vi "Set_valves.vi"() -> ()   [LabVIEW 2016]
panel:
  in  "Clean Cycle Wait Time (s)":u32=8
  in  "Clean Cycle":bool
  in  "Close all Valves":bool
  in  "Set new Values":bool
  in  "stop":bool
  in  "Update Immediately":bool=TRUE
  in  "Which box":string[](array[string])=["A", "B", "C"]
  in  "Channel Nums":string[](array[string])=["1", "2", "3", "4", "5", "6", "7", "8"]
  in  "Channels":bool[][](array[boolean])=[[FALSE, FALSE, FALSE], [FALSE, FALSE, FALSE], [FALSE, FALSE, FALSE], [FALSE, FALSE, FALSE], [FALSE, FALSE, FALSE], [FALSE, FALSE, FALSE], [FALSE, FALSE, FALSE], [FALSE, FALSE, FALSE]]
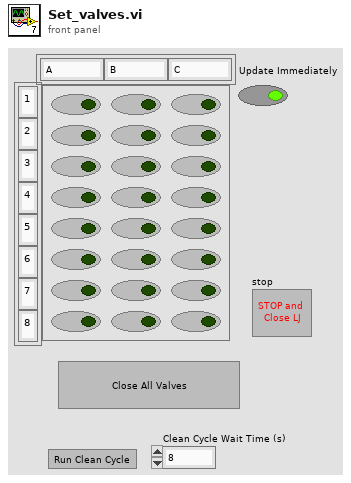
[diagram p1: front panel]
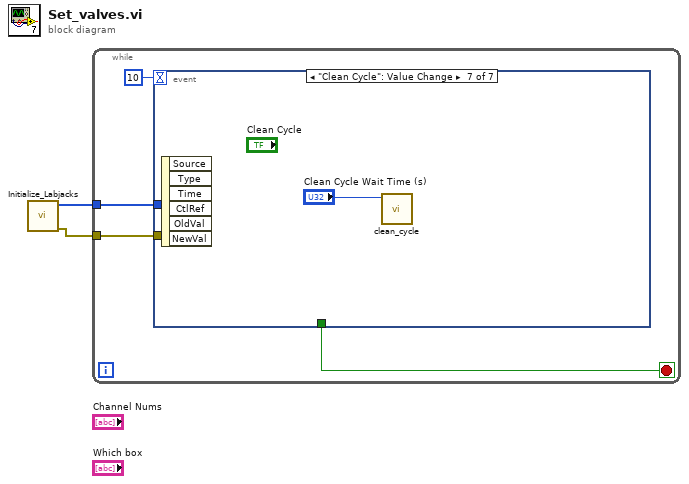
[diagram p0: block diagram]
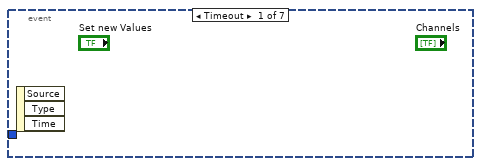
[diagram p2: hidden frame]
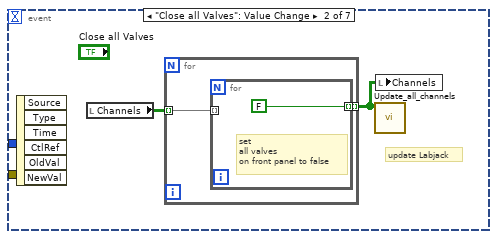
[diagram p3: hidden frame]
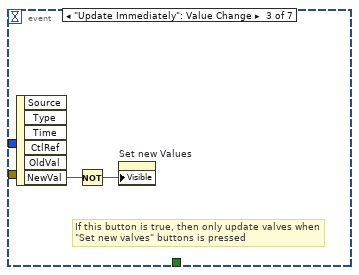
[diagram p4: hidden frame]
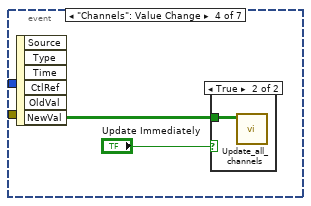
[diagram p5: hidden frame]
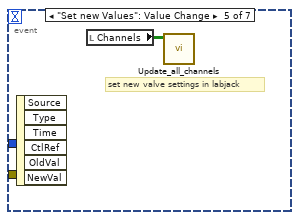
[diagram p7: hidden frame]
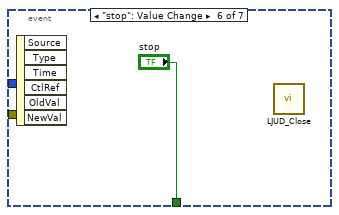
[diagram p8: hidden frame]
diagram:
  n1 = call "Initialize_Labjacks.vi"() -> ("error out"=w1:errorcluster, "LJ Handles"=w2:i32[])  [unwired: 10 in]
  n2 = while {
    tunnel: w2 -> [w3]
    tunnel: w1 -> [w4]
    stop <- w5 stop-if-true
    n3 = event shown="[6] \"Clean Cycle\": Value Change" {
      selector: _ -> [_ _ _ _ _ _ _]
      dyn-events: _ -> [_ _ _ _ _ _ _]
      timeout: 10 -> [_ _ _ _ _ _ _]
      tunnel: [_ _ _ _ _ "stop" _] -> w5
      tunnel: w4 -> [_ _ _ _ _ _ _]
      tunnel: w3 -> [_ _ _ _ _ _ _]
      event Timeout {
        n4 = event-data() -> ()  [unwired: 1 in, 3 out]
      }
      event "Close all Valves": Value Change {
        # "update Labjack"
        n5 = event-data() -> ()  [unwired: 1 in, 6 out]
        n6 = local read "Channels"() -> (w8:bool[][])
        n7 = for {
          tunnel: w8 -> [w10] mode=indexing
          tunnel: [w9] -> w7 mode=indexing
          n8 = for {
            tunnel: w10 -> [_] mode=indexing
            tunnel: [FALSE] -> w9 mode=indexing
            # "set\nall valves\non front panel to false"
          }
        }
        n9 = call "Update_all_channels.vi"("Channel Values"=w7) -> ()  [unwired: 11 in]
        n10 = local write "Channels"(w7) -> ()
      }
      event "Update Immediately": Value Change {
        # "If this button is true, then only update valves when\n\"Set new valves\" buttons is pressed"
        n11 = event-data() -> ("NewVal"=w13:bool)  [unwired: 1 in, 5 out]
        n12 = Not(x=w13) -> (.not. x?=w12:bool)
        n13 = property on="Set new Values" class="Bool (strict)"("Visible"=w12) -> ()  [unwired: 2 in, 2 out]
      }
      event "Channels": Value Change {
        n14 = event-data() -> ("NewVal"=w14:bool[][])  [unwired: 1 in, 5 out]
        n15 = case shown="True" "Update Immediately" {
          tunnel: w14 -> [_ w16]
          frame False {
          }
          frame True {
            n16 = call "Update_all_channels.vi"("Channel Values"=w16) -> ()  [unwired: 11 in]
          }
        }
      }
      event "Set new Values": Value Change {
        # "set new valve settings in labjack"
        n17 = event-data() -> ()  [unwired: 1 in, 6 out]
        n18 = local read "Channels"() -> (w17:bool[][])
        n19 = call "Update_all_channels.vi"("Channel Values"=w17) -> ()  [unwired: 11 in]
      }
      event "stop": Value Change {
        n20 = event-data() -> ()  [unwired: 1 in, 6 out]
        n21 = call "LJUD_Close.vi"() -> ()  [unwired: 11 in, 1 out]
      }
      event "Clean Cycle": Value Change {
        n22 = event-data() -> ()  [unwired: 1 in, 6 out]
        n23 = call "clean_cycle.vi"("seconds to wait"="Clean Cycle Wait Time (s)") -> ()  [unwired: 11 in]
      }
    }
  }
